vi "Create Reg Files.vi"(8 "void init_ios(void)":string, 9 "defines":string, 11 "path":path) -> (2 "app_regs.c":string, 3 "app_regs.h":string)   [LabVIEW 2010]
uses:
  read_excel_values.llb/GetXL_CellValues_2D_String.vi
panel:
  out "error out":errorcluster
  # "Type: U8, I8, U16, I16, U32, I32, U64, I64, FLOAT"
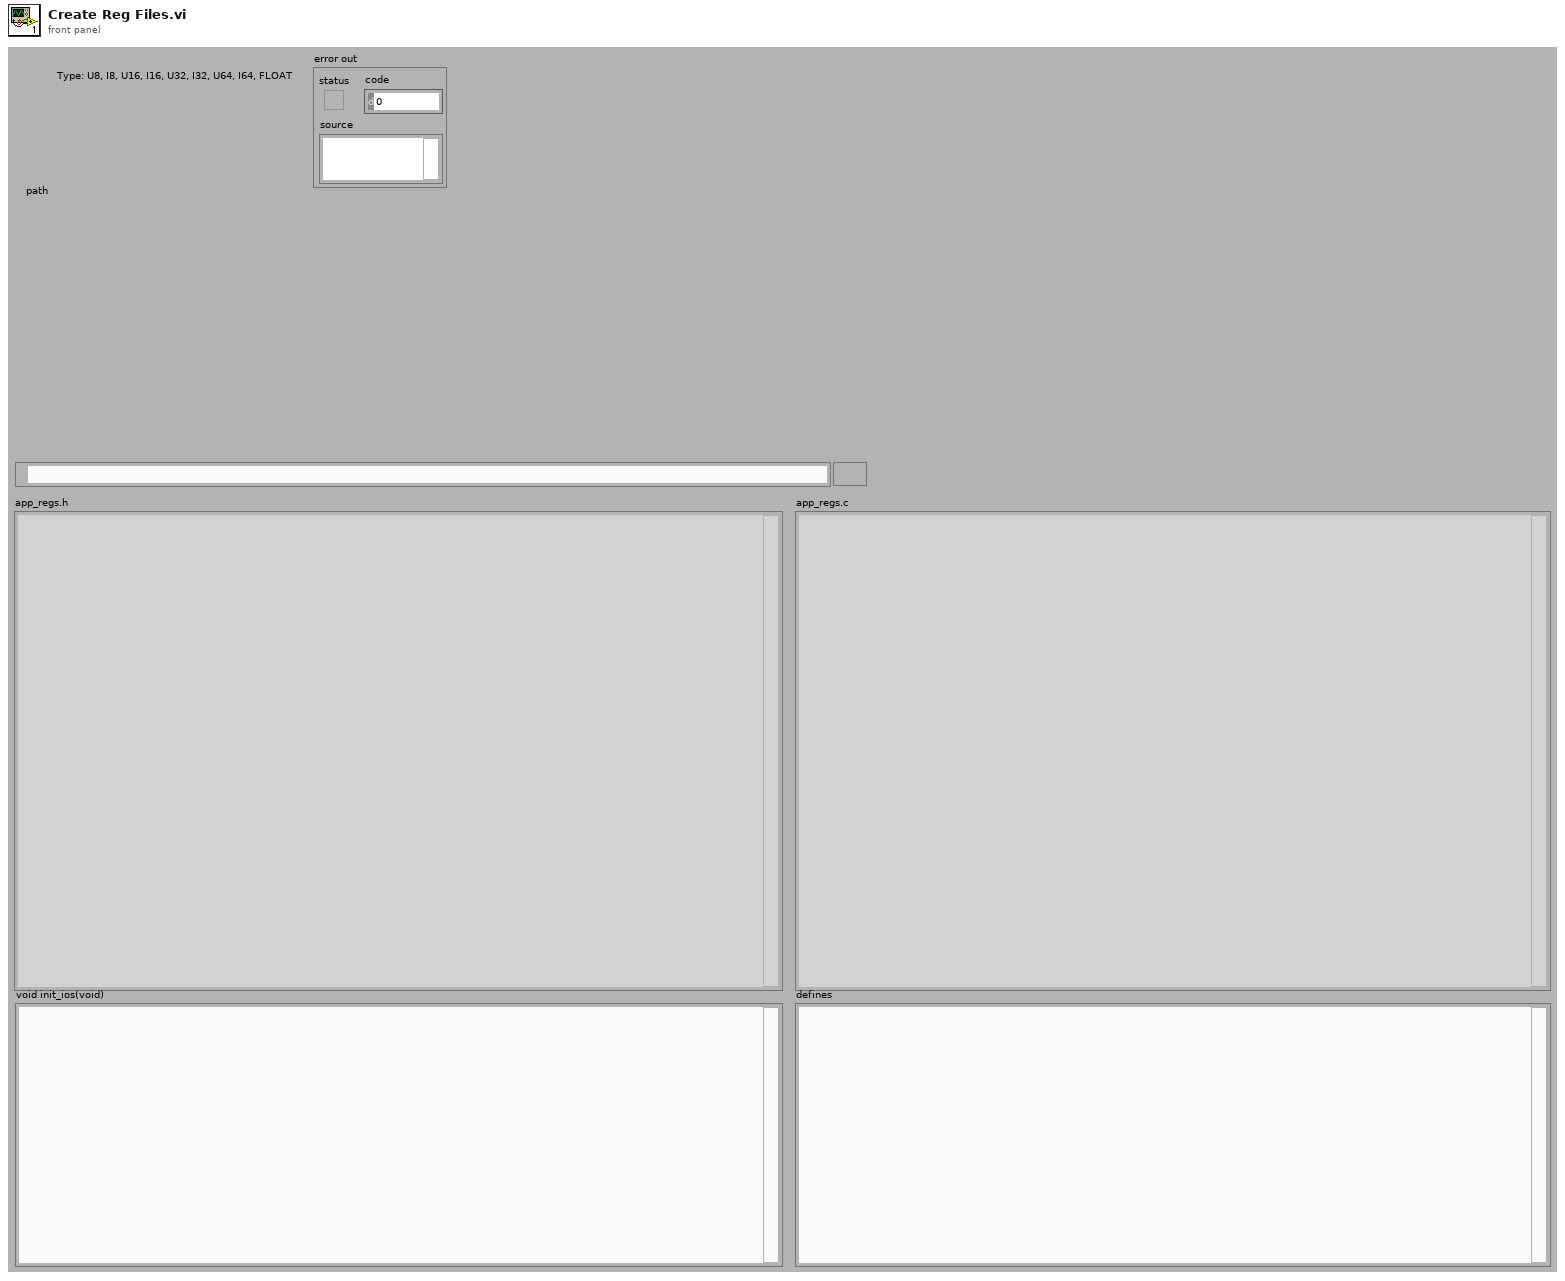
[diagram p1: front panel]
types:
  T1 = cluster{"Excel._Application":refnum<k7>, "Workbooks":refnum<k7>}
  T2 = cluster{"Excel._Application":refnum<k7>, "Workbooks":refnum<k7>, "Open":refnum<k7>}
  T3 = cluster{"Excel._Application":refnum<k7>, "Workbooks":refnum<k7>, "Open":refnum<k7>, "Worksheets":refnum<k7>, "Excel._Worksheet":refnum<k7>}
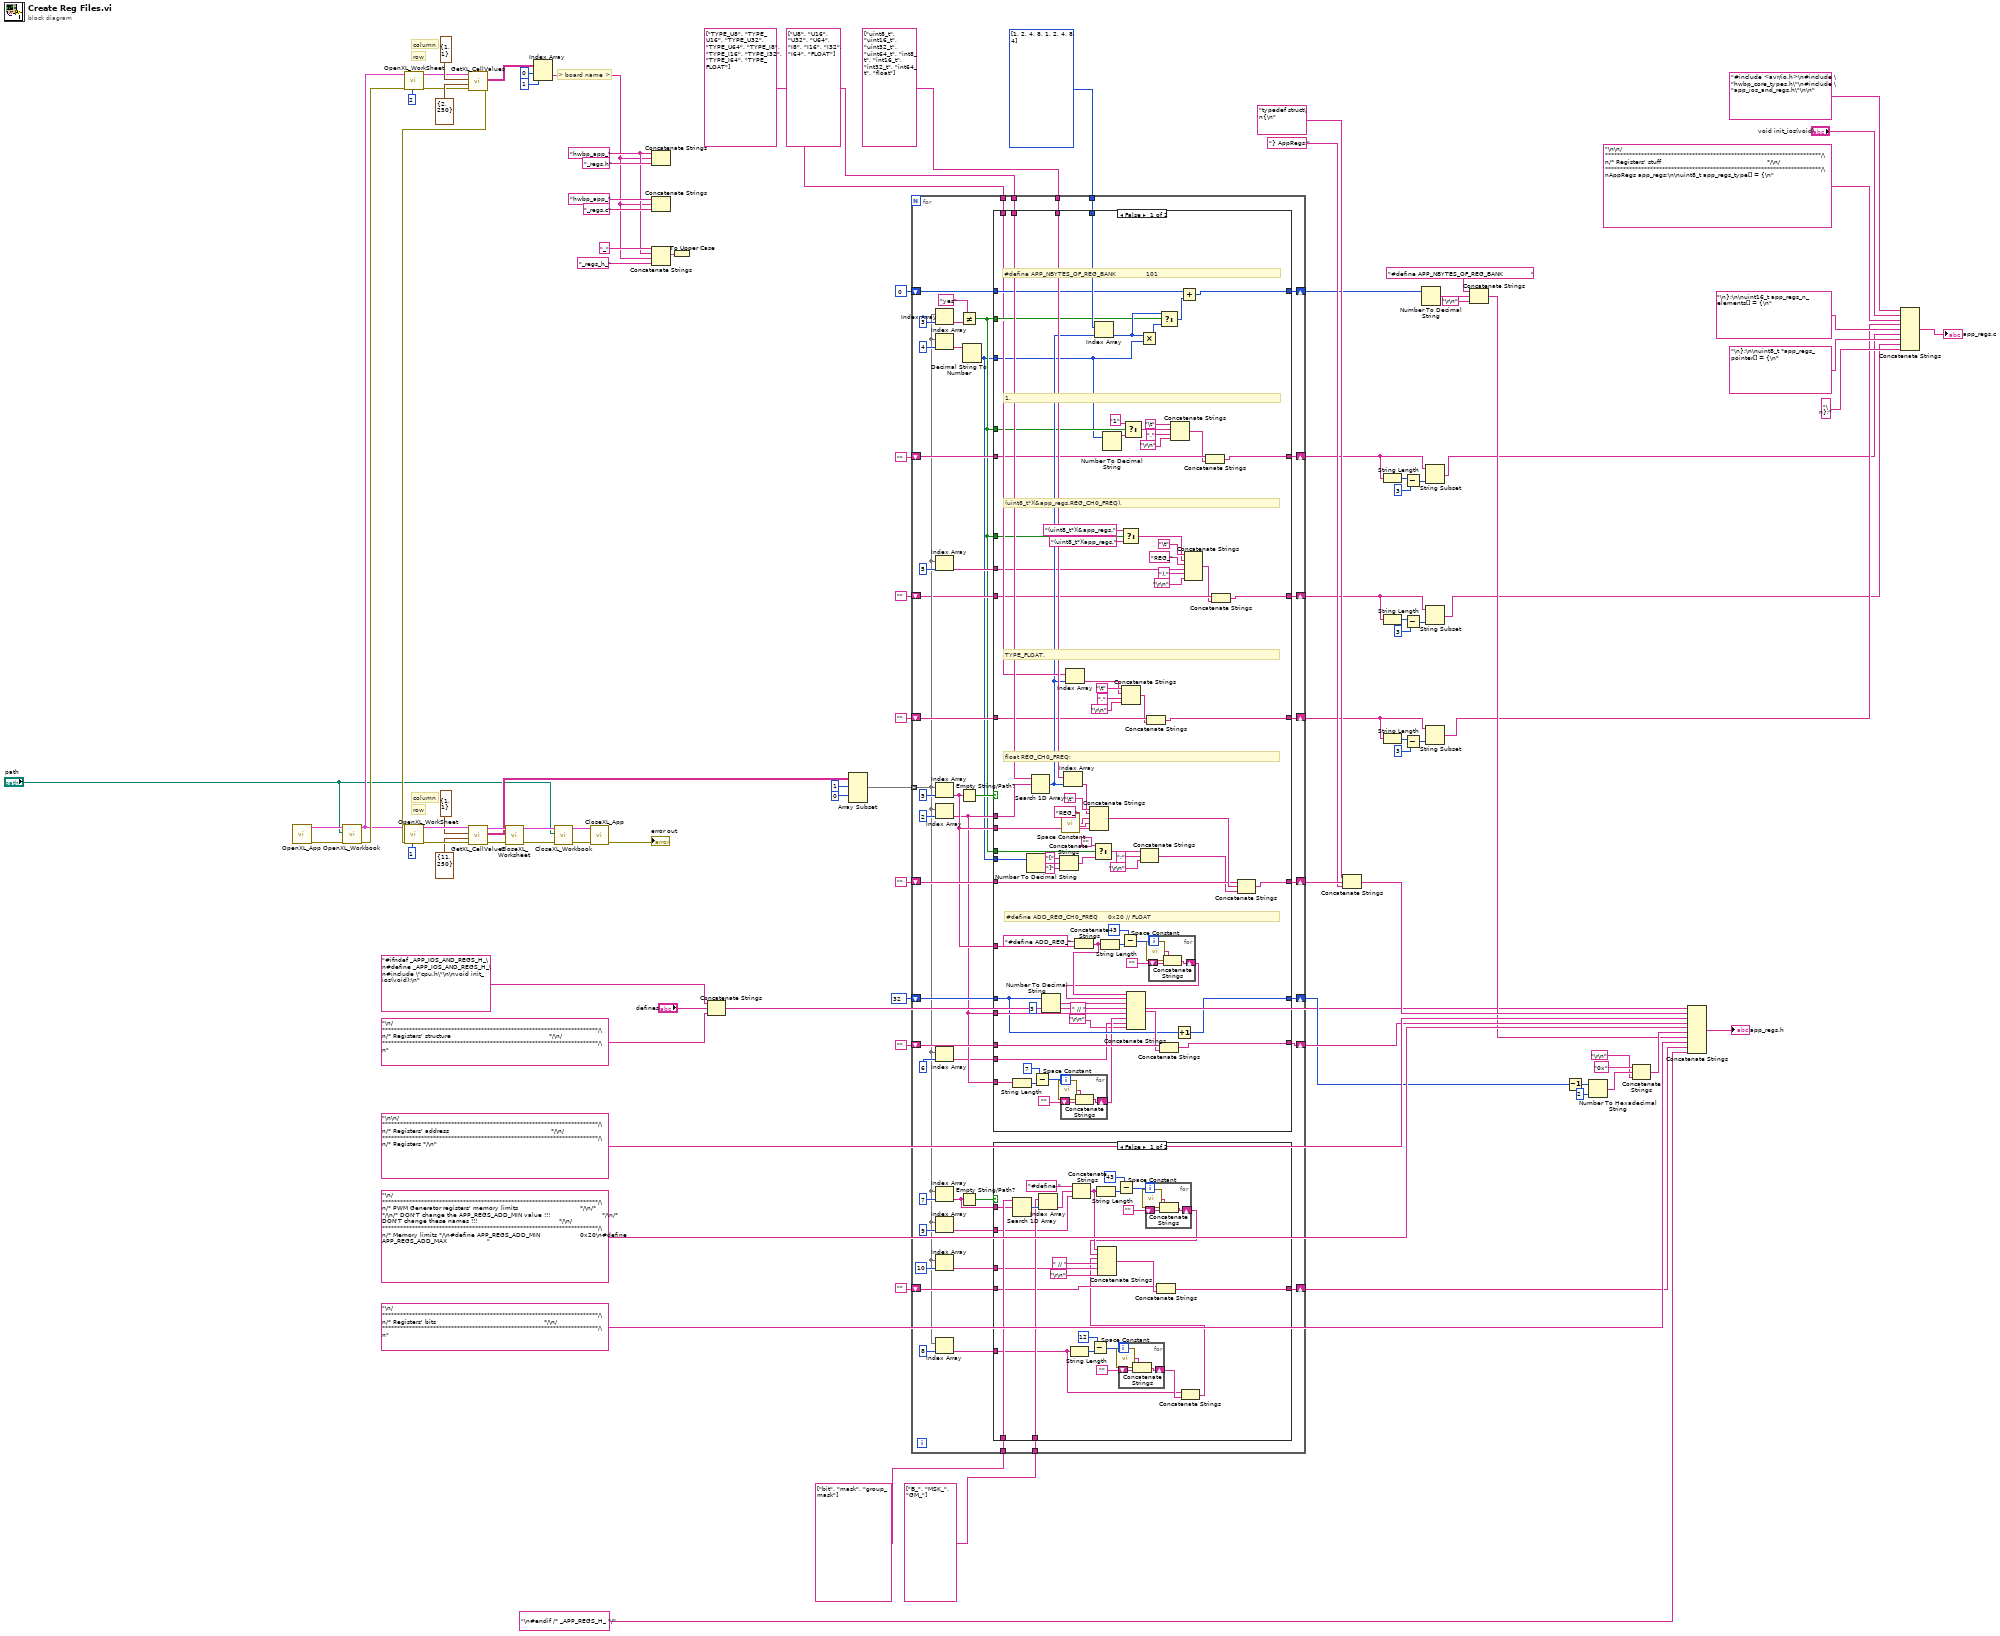
[diagram p0: block diagram]
diagram:
  w10 = "hwbp_app_" ("string")
  # "> board name >"
  # "row"
  # "column"
  # "row"
  # "column"
  n1 = call "OpenXL_App.vi"() -> ("error out"=w93:errorcluster, "Refnum Cluster"=w94:T1)  [unwired: 10 in]
  n2 = call "OpenXL_Workbook.vi"("error in"=w93, "path"="path", "Refnum Cluster In"=w94) -> ("error out"=w68:errorcluster, "Refnum Cluster Out"=w66:T2)  [unwired: 7 in]
  n3 = call "OpenXL_WorkSheet.vi"("Sheet"=2, "error in (no error)"=w68, "Refnum Cluster In"=w66) -> ("error out"=w70:errorcluster, "Refnum Cluster Out"=w69:T3)  [unwired: 7 in]
  n4 = call-poly "GetXL_CellValues.vi"("error in"=w70, "End"=cluster{"Column":i32, "Row":i32} {"Column"=2, "Row"=250}, "Start"=cluster{"Column":i32, "Row":i32} {"Column"=1, "Row"=1}, "Refnum Cluster In"=w69) -> ("error out"=w67:errorcluster, "data"=w63:string[][])  [unwired: 5 in, 1 out]
  n5 = call "OpenXL_WorkSheet.vi"("Sheet"=1, "error in (no error)"=w67, "Refnum Cluster In"=w66) -> ("error out"=w100:errorcluster, "Refnum Cluster Out"=w101:T3)  [unwired: 7 in]
  n6 = call-poly "GetXL_CellValues.vi"("error in"=w100, "End"=cluster{"Column":i32, "Row":i32} {"Column"=11, "Row"=250}, "Start"=cluster{"Column":i32, "Row":i32} {"Column"=1, "Row"=1}, "Refnum Cluster In"=w101) -> ("error out"=w91:errorcluster, "data"=w77:string[][], "Refnum Cluster Out"=w92:T3)  [unwired: 5 in]
  n7 = call "CloseXL_Worksheet.vi"("error in (no error)"=w91, "Refnum Cluster In"=w92) -> ("error out"=w89:errorcluster, "Refnum Cluster Out"=w90:T2)  [unwired: 8 in]
  n8 = Index Array(array=w63, index (row)=0, index (col)=1 ("disabled index (col)")) -> (element=w9:string)
  n9 = call "CloseXL_Workbook.vi"("error in (no error)"=w89, "path"="path", "Refnum Cluster In"=w90) -> ("error out"=w98:errorcluster, "Refnum Cluster Out"=w99:T1)  [unwired: 7 in]
  n10 = call "CloseXL_App.vi"("error in (no error)"=w98, "Refnum Cluster In"=w99) -> ("error out"=→"error out":errorcluster)  [unwired: 9 in]
  n11 = Concatenate Strings(w10, w9, "_regs.h" ("string")) -> ()  [unwired: 1 out]
  n12 = Concatenate Strings("hwbp_app_" ("string"), w9, "_regs.c" ("string")) -> ()  [unwired: 1 out]
  n13 = Concatenate Strings("_" ("string"), w10, w9, "_regs_h_" ("string")) -> (w12:string)
  n14 = To Upper Case(1:w12) -> ()  [unwired: 1 out]
  n15 = Concatenate Strings("#ifndef _APP_IOS_AND_REGS_H_\n#define _APP_IOS_AND_REGS_H_\n#include \"cpu.h\"\n\nvoid init_ios(void);\n" ("string"), "defines", "\n/************************************************************************/\n/* Registers' structure                                                 */\n/************************************************************************/\n" ("string")) -> (w6:string)
  n16 = Array Subset(array=w77, index (row)=1 ("index"), index (col)=0 ("index")) -> (w74:string[][])  [unwired: 2 in]
  n17 = for {
    tunnel: w74 -> [w107] mode=indexing
    tunnel: string[] ["U8", "U16", "U32", "U64", "I8", "I16", "I32", "I64", "FLOAT"] -> [w146]
    tunnel: string[] ["uint8_t", "uint16_t", "uint32_t", "uint64_t", "int8_t", "int16_t", "int32_t", "int64_t", "float"] -> [w145]
    shift-right: [w143] -> w80
    shift-left: "" -> [w144]
    shift-right: [w140] -> w54
    shift-left: 32 ("x") -> [w141]
    shift-right: [w138] -> w59
    shift-left: "" -> [w139]
    tunnel: i32[] [1, 2, 4, 8, 1, 2, 4, 8, 4] -> [w137]
    shift-right: [w136] -> w48
    shift-left: 0 ("x") -> [w135]
    tunnel: string[] ["bit", "mask", "group_mask"] -> [w125]
    tunnel: string[] ["B_", "MSK_", "GM_"] -> [w123]
    shift-right: [w118] -> w39
    shift-left: "" -> [w116]
    tunnel: string[] ["TYPE_U8", "TYPE_U16", "TYPE_U32", "TYPE_U64", "TYPE_I8", "TYPE_I16", "TYPE_I32", "TYPE_I64", "TYPE_FLOAT"] -> [w113]
    shift-right: [w112] -> w28
    shift-left: "" -> [w111]
    shift-right: [w109] -> w19
    shift-left: "" -> [w110]
    shift-right: [w104] -> w17
    shift-left: "" -> [w105]
    n18 = Index Array(array=w107, index=3) -> (element=w133:string)
    n19 = Index Array(array=w107, index=4) -> (element=w130:string)
    n20 = Index Array(array=w107, index=5) -> (element=w106:string)
    n21 = Index Array(array=w107, index=5) -> (element=w142:string)
    n22 = Index Array(array=w107, index=2) -> (element=w128:string)
    n23 = Index Array(array=w107, index=6) -> (element=w127:string)
    n24 = Index Array(array=w107, index=7) -> (element=w124:string)
    n25 = Index Array(array=w107, index=9) -> (element=w120:string)
    n26 = Index Array(array=w107, index=10) -> (element=w119:string)
    n27 = Index Array(array=w107, index=8) -> (element=w114:string)
    n28 = Not Equal?(x="yes", y=w133) -> (x != y?=w103:bool)
    n29 = Empty String/Path?(string/path=w142) -> (empty?=w148:bool)
    n30 = Empty String/Path?(string/path=w124) -> (empty?=w117:bool)
    n31 = Decimal String To Number(string=w130) -> (number=w102:i32)  [unwired: 2 in, 1 out]
    n32 = case shown="False" w148 {
      tunnel: w128 -> [w268 _]
      tunnel: w146 -> [w267 _]
      tunnel: w145 -> [w266 _]
      tunnel: w142 -> [w261 _]
      tunnel: w144 -> [w264 w281]
      tunnel: [w263 w281] -> w143
      tunnel: w142 -> [w260 _]
      tunnel: w141 -> [w245 w280]
      tunnel: w128 -> [w250 _]
      tunnel: [w246 w280] -> w140
      tunnel: w139 -> [w249 w279]
      tunnel: [w247 w279] -> w138
      tunnel: w137 -> [w244 _]
      tunnel: [w242 w278] -> w136
      tunnel: w135 -> [w243 w278]
      tunnel: w103 -> [w238 _]
      tunnel: w102 -> [w216 _]
      tunnel: w128 -> [w233 _]
      tunnel: w127 -> [w231 _]
      tunnel: w113 -> [w229 _]
      tunnel: w111 -> [w222 w277]
      tunnel: [w223 w277] -> w112
      tunnel: w103 -> [w220 _]
      tunnel: w110 -> [w212 w276]
      tunnel: [w211 w276] -> w109
      tunnel: w103 -> [w202 _]
      tunnel: w106 -> [w199 _]
      tunnel: w105 -> [w196 w275]
      tunnel: [w195 w275] -> w104
      tunnel: w103 -> [w190 _]
      tunnel: w102 -> [w189 _]
      frame False {
        # "1,"
        # "(uint8_t*)(&app_regs.REG_CH0_FREQ),"
        # "TYPE_FLOAT,"
        # "#define APP_NBYTES_OF_REG_BANK               101"
        # "float\tREG_CH0_FREQ;"
        # "#define ADD_REG_CH0_FREQ\t\t\t\t\t0x20\t// FLOAT"
        n33 = String Length(string=w233) -> (length=w234:i32)
        n34 = Number To Decimal String(number=w189) -> (decimal integer string=w188:string)  [unwired: 1 in]
        n35 = Search 1D Array(1D array=w267, element=w268) -> (index of element=w228:i32)  [unwired: 1 in]
        n36 = Subtract(x=7, y=w234) -> (x-y=w236:i32)
        n37 = Number To Decimal String(number=w245, width (-)=i16 3) -> (decimal integer string=w253:string)
        n38 = Concatenate Strings("[" ("string"), w188, "]" ("string")) -> (w185:string)
        n39 = for {
          N: w236 -> [_]
          shift-right: [w269] -> w232
          shift-left: "" -> [w271]
          n40 = call <vilib>:"Space Constant.vi"() -> ("String"=w270:string)
          n41 = Concatenate Strings(w270, w271) -> (w269:string)
        }
        n42 = call <vilib>:"Space Constant.vi"() -> ("String"=w206:string)
        n43 = Index Array(array=w266, index=w228) -> (element=w207:string)
        n44 = Index Array(array=w229, index=w228) -> (element=w226:string)
        n45 = Concatenate Strings("#define ADD_REG_" ("string"), w260) -> (w255:string)
        n46 = Concatenate Strings("\t", w207, w206, "REG_" ("string"), w261) -> (w265:string)
        n47 = Select(t="" ("x"), s=w190, f=w185) -> (s? t:f=w192:string)
        n48 = Index Array(array=w244, index=w228) -> (element=w239:i32)
        n49 = String Length(string=w255) -> (length=w259:i32)
        n50 = Number To Decimal String(number=w216) -> (decimal integer string=w214:string)  [unwired: 1 in]
        n51 = Subtract(x=43, y=w259) -> (x-y=w257:i32)
        n52 = Select(t="(uint8_t*)(&app_regs." ("string"), s=w202, f="(uint8_t*)(app_regs." ("string")) -> (s? t:f=w201:string)
        n53 = Concatenate Strings("\t", w226, "," ("string"), "\r\n") -> (w221:string)
        n54 = Select(t="1" ("x"), s=w220, f=w214) -> (s? t:f=w213:string)
        n55 = Multiply(x=w239, y=w216) -> (x*y=w240:i32)
        n56 = Concatenate Strings(w192, ";" ("string"), "\r\n") -> (w183:string)
        n57 = Concatenate Strings(w222, w221) -> (w223:string)
        n58 = for {
          N: w257 -> [_]
          shift-right: [w272] -> w254
          shift-left: "" -> [w274]
          n59 = call <vilib>:"Space Constant.vi"() -> ("String"=w273:string)
          n60 = Concatenate Strings(w273, w274) -> (w272:string)
        }
        n61 = Concatenate Strings(w255, w254, w253, " // " ("string"), w250, w232, w231, "\r\n") -> (w248:string)
        n62 = Concatenate Strings(w249, w248) -> (w247:string)
        n63 = Select(t=w239, s=w238, f=w240) -> (s? t:f=w241:i32)
        n64 = Concatenate Strings("\t", w213, "," ("string"), "\r\n") -> (w210:string)
        n65 = Increment(x=w245) -> (x+1=w246:i32)
        n66 = Add(x=w243, y=w241) -> (x+y=w242:i32)
        n67 = Concatenate Strings("\t", w201, "REG_" ("string"), w199, ")," ("string"), "\r\n") -> (w194:string)
        n68 = Concatenate Strings(w212, w210) -> (w211:string)
        n69 = Concatenate Strings(w196, w194) -> (w195:string)
        n70 = Concatenate Strings(w264, w265, w183) -> (w263:string)
      }
      frame True {
      }
    }
    n71 = case shown="False" w117 {
      tunnel: w125 -> [w174 _]
      tunnel: w124 -> [w173 _]
      tunnel: w123 -> [w172 _]
      tunnel: w120 -> [w162 _]
      tunnel: w119 -> [w161 _]
      tunnel: [w159 w182] -> w118
      tunnel: w116 -> [w158 w182]
      tunnel: w114 -> [w151 _]
      frame False {
        n72 = Search 1D Array(1D array=w174, element=w173) -> (index of element=w175:i32)  [unwired: 1 in]
        n73 = Index Array(array=w172, index=w175) -> (element=w167:string)
        n74 = String Length(string=w151) -> (length=w153:i32)
        n75 = Concatenate Strings("#define " ("string"), w167, w162) -> (w165:string)
        n76 = Subtract(x=12, y=w153) -> (x-y=w155:i32)
        n77 = String Length(string=w165) -> (length=w171:i32)
        n78 = Subtract(x=43, y=w171) -> (x-y=w169:i32)
        n79 = for {
          N: w155 -> [_]
          shift-right: [w176] -> w152
          shift-left: "" -> [w178]
          n80 = call <vilib>:"Space Constant.vi"() -> ("String"=w177:string)
          n81 = Concatenate Strings(w177, w178) -> (w176:string)
        }
        n82 = for {
          N: w169 -> [_]
          shift-right: [w179] -> w164
          shift-left: "" -> [w181]
          n83 = call <vilib>:"Space Constant.vi"() -> ("String"=w180:string)
          n84 = Concatenate Strings(w180, w181) -> (w179:string)
        }
        n85 = Concatenate Strings(w151, w152) -> (w150:string)
        n86 = Concatenate Strings(w165, w164, w150, " // " ("string"), w161, "\r\n") -> (w160:string)
        n87 = Concatenate Strings(w158, w160) -> (w159:string)
      }
      frame True {
      }
    }
  }
  n88 = Concatenate Strings("typedef struct\n{\n" ("string"), w80, "} AppRegs;" ("string")) -> (w78:string)
  n89 = String Length(string=w19) -> (length=w23:i32)
  n90 = String Length(string=w17) -> (length=w24:i32)
  n91 = String Length(string=w28) -> (length=w31:i32)
  n92 = Subtract(x=w23, y=3 ("index")) -> (x-y=w21:i32)
  n93 = Subtract(x=w24, y=3 ("index")) -> (x-y=w26:i32)
  n94 = Subtract(x=w31, y=3 ("index")) -> (x-y=w29:i32)
  n95 = Number To Decimal String(number=w48) -> (decimal integer string=w45:string)  [unwired: 1 in]
  n96 = String Subset(string=w19, length (rest)=w21) -> (substring=w20:string)  [unwired: 1 in]
  n97 = String Subset(string=w17, length (rest)=w26) -> (substring=w18:string)  [unwired: 1 in]
  n98 = String Subset(string=w28, length (rest)=w29) -> (substring=w27:string)  [unwired: 1 in]
  n99 = Concatenate Strings("#define APP_NBYTES_OF_REG_BANK              " ("string"), w45, "\r\n") -> (w44:string)
  n100 = Decrement(x=w54) -> (x-1=w53:i32)
  n101 = Number To Hexadecimal String(1:i16 2 ("width (-)"), 2:w53) -> (0:w55:string)
  n102 = Concatenate Strings("0x" ("string"), w55, "\r\n") -> (w52:string)
  n103 = Concatenate Strings(w6, w78, "\n\n/************************************************************************/\n/* Registers' address                                                   */\n/************************************************************************/\n/* Registers */\n" ("string"), w59, "\n/************************************************************************/\n/* PWM Generator registers' memory limits                               */\n/*                                                                      */\n/* DON'T change the APP_REGS_ADD_MIN value !!!                          */\n/* DON'T change these names !!!                                         */\n/************************************************************************/\n/* Memory limits */\n#define APP_REGS_ADD_MIN                    0x20\n#define APP_REGS_ADD_MAX                    " ("string"), w52, w44, "\n/************************************************************************/\n/* Registers' bits                                                      */\n/************************************************************************/\n" ("string"), w39, "\n#endif /* _APP_REGS_H_ */" ("string")) -> (→"app_regs.h":string)
  n104 = Concatenate Strings("#include <avr/io.h>\n#include \"hwbp_core_types.h\"\n#include \"app_ios_and_regs.h\"\n\n" ("string"), "void init_ios(void)", "\n\n/************************************************************************/\n/* Registers' stuff                                                     */\n/************************************************************************/\nAppRegs app_regs;\n\nuint8_t app_regs_type[] = {\n" ("string"), w27, "\n};\n\nuint16_t app_regs_n_elements[] = {\n" ("string"), w20, "\n};\n\nuint8_t *app_regs_pointer[] = {\n" ("string"), w18, "\n};" ("string")) -> (→"app_regs.c":string)
